vi "Server - Main.vi"(8 "error in (no error)":errorcluster) -> (0 "error out":errorcluster)   [LabVIEW 2019]
doc: "This VI runs on the server."
panel:
  out "log file path":path
  out "log file name":string
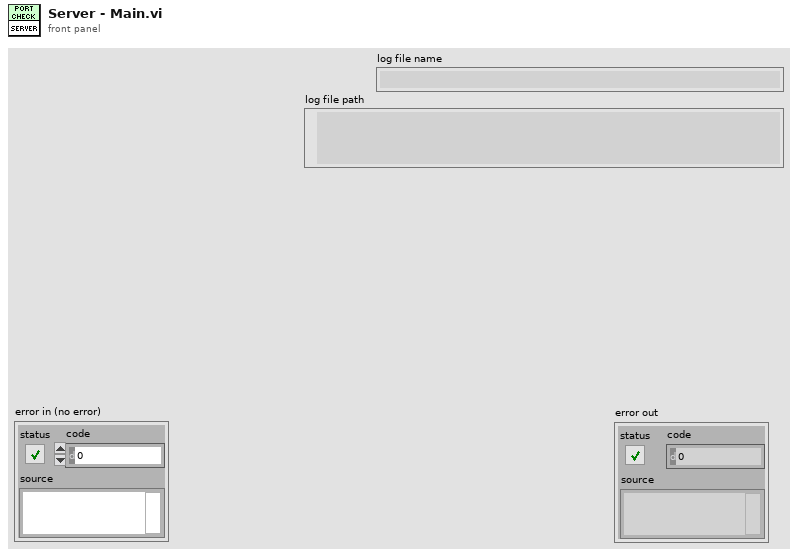
[diagram p1: front panel]
types:
  T1 = typedef "Ports to Check.ctl" = cluster{"TCP Ports":u16[], "UDP Ports":u16[]}
  T2 = typedef "Results.ctl" = T3[]
  T3 = typedef "log data cluster.ctl" = cluster{"Time Stamp":timestamp, "Port Number":u16, "Communication Type":T4, "success?":bool, "error in":errorcluster}
  T4 = typedef "Communication Types.ctl" = enum16{"UDP - Server to Client", "UDP - Client to Server", "TCP - Server to Client", "TCP - Client to Server"}
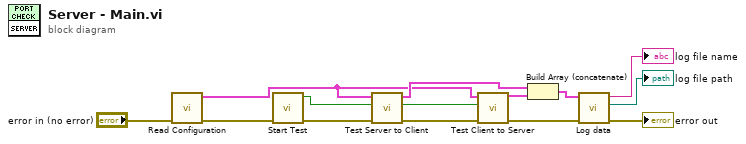
[diagram p0: block diagram]
diagram:
  n1 = call "Read Configuration.vi"("error in (no error)"="error in (no error)") -> ("error out"=w13:errorcluster, "Ports to Check"=w2:T1)  [unwired: 9 in]
  n2 = call "Start Test.vi"("error in (no error)"=w13) -> ("error out"=w11:errorcluster, "Connection Established?"=w10:bool)  [unwired: 9 in]
  n3 = call "Test Server to Client.vi"("Ports to Check"=w2, "Connection Established?"=w10, "error in (no error)"=w11) -> ("Results"=w9:T2, "Test Finished?"=w3:bool, "error out"=w5:errorcluster)  [unwired: 5 in]
  n4 = call "Test Client to Server.vi"("Ports to Check"=w2, "Connection Established?"=w3, "error in (no error)"=w5) -> ("Results"=w1:T2, "error out"=w4:errorcluster)  [unwired: 5 in, 1 out]
  n5 = Build Array (concatenate)(w9, w1) -> (w8:T2)
  n6 = call "Log data.vi"("error in (no error)"=w4, "Results"=w8) -> ("error out"=→"error out":errorcluster, "log file path"=→"log file path":path, "log file name"=→"log file name":string)  [unwired: 7 in]
